vi "isExisting.vi"(2 "error in (no error)":errorcluster, 3 "name":string) -> (0 "error out":errorcluster, 1 "obj exists":bool)   [LabVIEW 2012, in "HGF_ObjectManager.lvlib"]
doc: "This VI checks whether an object exists or not."
uses:
  HGF_ObjectManager.lvlib
  action.ctl
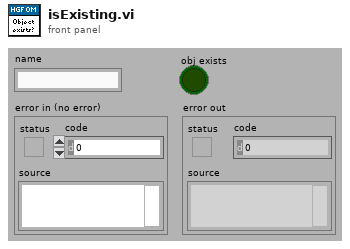
[diagram p1: front panel]
types:
  T1 = typedef "HGF_ObjectManager.lvlib/action.ctl" = enum16{"add", "remove", "name2ref", "ref2name ", "obj exists?", "cleanup", "get object list", "reset"}
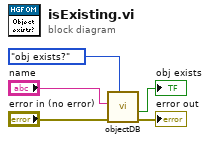
[diagram p0: block diagram]
diagram:
  n1 = call "objectDB.vi"("Action"=action."obj exists?", "error in (no error)"="error in (no error)", "name"="name") -> ("error out"=→"error out":errorcluster, "obj exists"=→"obj exists":bool)  [unwired: 2 in, 5 out]
